vi "Create.vi"(10 "Value":string) -> (3 "StringValue out":refnum<class "StringValue.lvclass">)   [LabVIEW 2020, in "Futures-Examples.lvlib" / "StringValue.lvclass"]
uses:
  StringValue.lvclass
  StringValue.lvclass/StringValue.ctl
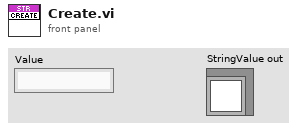
[diagram p1: front panel]
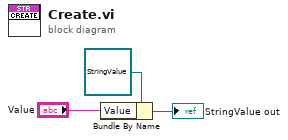
[diagram p0: block diagram]
diagram:
  n1 = Bundle By Name(cluster=refnum<class "StringValue.lvclass"> refnum ("StringValue in"), "Value"="Value") -> (→"StringValue out":refnum<class "StringValue.lvclass">)
